vi "未命名 1.vi"   [LabVIEW 2015]
uses:
  Public/DMM/Victor8246/Victor8246.lvlib
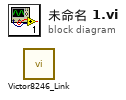
[diagram p0: block diagram]
diagram:
  n1 = call "Victor8246_Link.vi"() -> ()  [unwired: 6 in, 2 out]
